vi "Get Simulated Active DTCs.vi"(8 "error in (no error)":errorcluster, 10 "Address":u8, 11 "Simulated Addresses LUT":variant) -> (0 "error out":errorcluster, 1 "DTC Frame":u8[](array[numeric]), 2 "# of Enabled":u8, 3 "Address found":bool)   [LabVIEW 2013, in "J1939 Addon Engine.lvlib"]
uses:
  J1939 Addon Engine.lvlib
  Types/Simulated Settings.ctl
  Shared/Types/Compiled Simulated Settings.ctl
  Shared/Types/Monitor Settings.ctl
  <vilib>/NI Veristand/Custom Device API/Block Data Reference.ctl
  <vilib>/NI Veristand/Custom Device API/Data Reference.ctl
  Types/DTC FIFOs.ctl
  <vilib>/NI Veristand/Custom Device API/Custom Device API.lvlib
  Shared/J1939 Addon Shared.lvlib
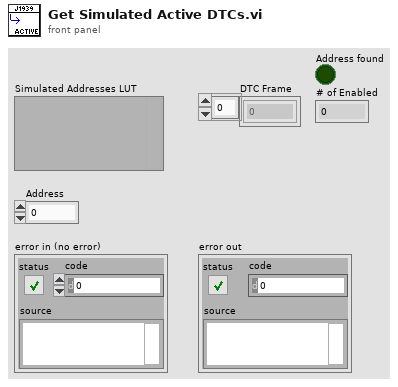
[diagram p1: front panel]
types:
  T1 = typedef "J1939 Addon Engine.lvlib/Simulated Settings.ctl" = cluster{"Simulated Addresses":T2, "FIFOs":T6}
  T2 = typedef "J1939 Addon Shared.lvlib/Compiled Simulated Settings.ctl" = cluster{"J1939 XNET Settings":T3, "DM1 Data":T4[], "DM1 Data":dbl[], "DM1 Enable?":T4[], "DM1 Enable?":dbl[], "DM2 Data":T4[], "DM2 Data":dbl[], "DM2 Enable?":T4[], "DM2 Enable?":dbl[]}
  T3 = typedef "J1939 Addon Shared.lvlib/Monitor Settings.ctl" = cluster{"J1939 Network Address":u8, "Name":u64}
  T4 = typedef "Custom Device API.lvlib/Block Data Reference.ctl" = cluster{"Data Reference":T5, "Offset":i32, "Length":i32}
  T5 = typedef "Custom Device API.lvlib/Data Reference.ctl" = i32
  T6 = typedef "J1939 Addon Engine.lvlib/DTC FIFOs.ctl" = cluster{"DM1 Data":refnum<k33>, "DM1 Enable?":refnum<k33>, "DM2 Data":refnum<k33>, "DM2 Enable?":refnum<k33>, "DM1 Reset?":refnum<k33>, "DM2 Reset?":refnum<k33>}
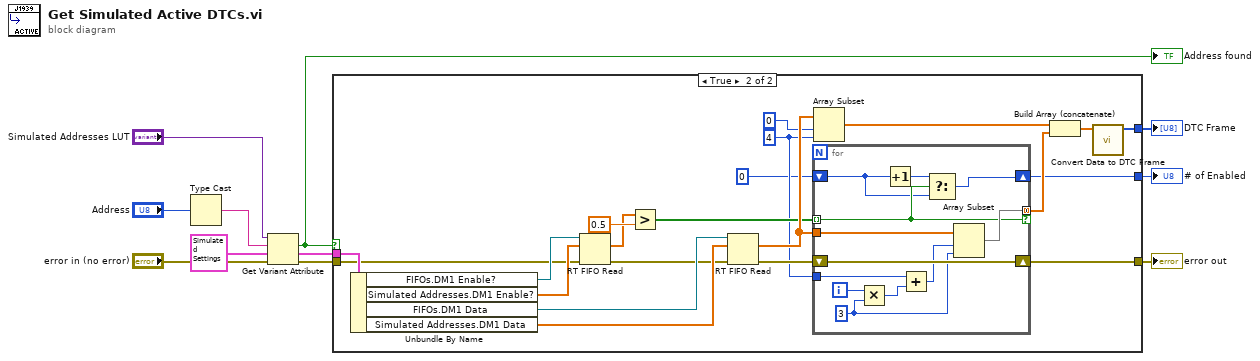
[diagram p0: block diagram]
diagram:
  n1 = Type Cast(x="Address") -> (*(type *) &x=w7:string)  [unwired: 1 in]
  n2 = Get Variant Attribute(Variant="Simulated Addresses LUT", name=w7, default value (empty Variant)=T1 {"Simulated Addresses"={"J1939 XNET Settings"={"J1939 Network Address"=0, "Name"=0}, "DM1 Data"=[], "DM1 Data"=[], "DM1 Enable?"=[], "DM1 Enable?"=[], "DM2 Data"=[], "DM2 Data"=[], "DM2 Enable?"=[], "DM2 Enable?"=[]}, "FIFOs"={"DM1 Data"=refnum, "DM1 Enable?"=refnum, "DM2 Data"=refnum, "DM2 Enable?"=refnum, "DM1 Reset?"=refnum, "DM2 Reset?"=refnum}} ("Cluster"), error in="error in (no error)") -> (found=w2:bool, value=w11:T1, error out=w10:errorcluster)  [unwired: 1 out]
  "Address found" <- w2
  n3 = case shown="True" w2 {
    tunnel: w11 -> [_ w26]
    tunnel: w10 -> [w12 w25]
    tunnel: [w12 w23] -> w4
    tunnel: [_ w17] -> w3
    tunnel: [_ w13] -> w1
    frame False {
    }
    frame True {
      w16 = 4 ("length")
      n4 = Unbundle By Name(w26) -> ("FIFOs.DM1 Enable?"=w27:refnum<k33>, "Simulated Addresses.DM1 Enable?"=w28:dbl[], "FIFOs.DM1 Data"=w29:refnum<k33>, "Simulated Addresses.DM1 Data"=w30:dbl[])
      n5 = RT FIFO Read(0:w27, 1:w28, 3:w25) -> (9:w19:dbl[], 11:w18:errorcluster)  [unwired: 1 in, 3 out]
      n6 = Greater?(x=w19, y=0.5) -> (0:w21:bool[])
      n7 = RT FIFO Read(0:w29, 1:w30, 3:w18) -> (9:w32:dbl[], 11:w22:errorcluster)  [unwired: 1 in, 3 out]
      n8 = for {
        tunnel: w21 -> [w37] mode=indexing
        shift-right: [w45] -> w23
        shift-left: w22 -> [w45]
        tunnel: w32 -> [w44]
        tunnel: [w43] -> w33 mode=concatenating if=w37
        tunnel: w16 -> [w40]
        shift-right: [w34] -> w13
        shift-left: u8 0 -> [w35]
        i -> [w42]
        w38 = 3 ("x")
        n9 = Multiply(x=w42, y=w38) -> (x*y=w41:i32)
        n10 = Increment(x=w35) -> (x+1=w36:u8)
        n11 = Add(x=w40, y=w41) -> (x+y=w39:i32)
        n12 = Select(t=w36, s=w37, f=w35) -> (s? t:f=w34:u8)
        n13 = Array Subset(array=w44, index=w39, length=w38) -> (w43:dbl[])
      }
      n14 = Array Subset(array=w32, index=0, length=w16) -> (w31:dbl[])
      n15 = Build Array (concatenate)(w31, w33) -> (w24:dbl[])
      n16 = call "Convert Data to DTC Frame.vi"("Data"=w24) -> ("DTC Frame"=w17:u8[])  [unwired: 10 in]
    }
  }
  "error out" <- w4
  "DTC Frame" <- w3
  "# of Enabled" <- w1
